vi "SetRelativePositionUm.vi"(8 "error in (no error)":errorcluster, 9 "RelativeMoveum":dbl min=0.0 max=200.0, 10 "Stage Label":string, 11 "Stage_MadCityLabMicro in":refnum<class "Stage_MadCityLabMicro.lvclass">) -> (0 "error out":errorcluster, 3 "Stage_MadCityLabMicro out":refnum<class "Stage_MadCityLabMicro.lvclass">)   [LabVIEW 2020, in "Stage_MadCityLabMicro.lvlib" / "Stage_MadCityLabMicro.lvclass"]
uses:
  Stage_MadCityLabMicro.lvclass
  Stage_MadCityLabMicro.lvclass/Stage_MadCityLabMicro.ctl
  Hardware Abstraction Layer/Component/Stage/Stage/Stage.lvclass
  Dependency/MicroDrive.dll
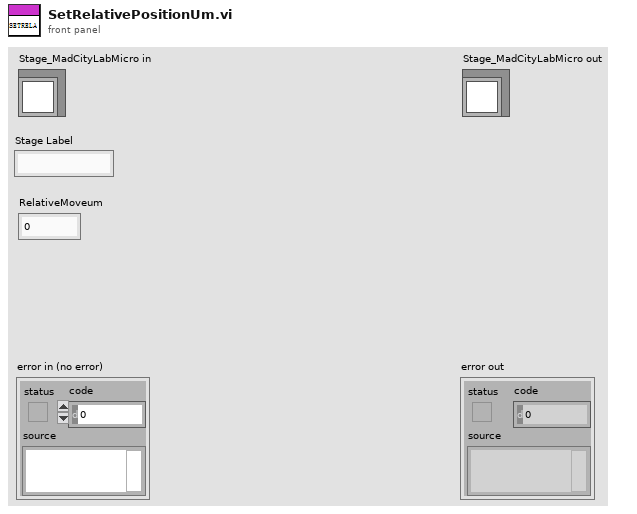
[diagram p1: front panel]
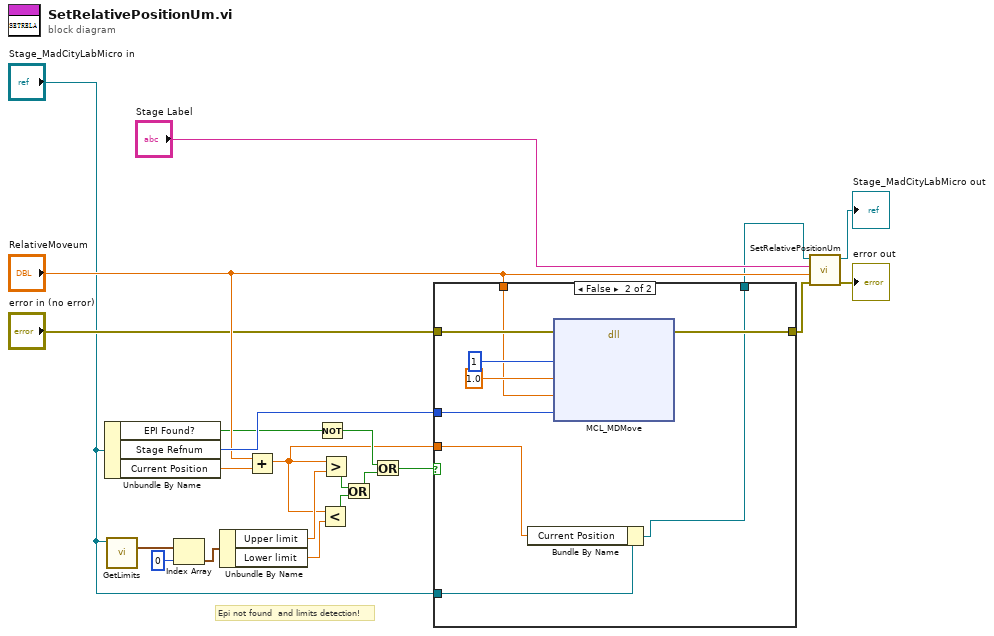
[diagram p0: block diagram]
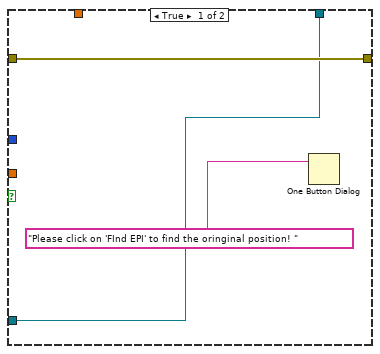
[diagram p2: hidden frame]
diagram:
  # "Epi not found  and limits detection!"
  n1 = Unbundle By Name("Stage_MadCityLabMicro in") -> ("EPI Found?"=w6:bool, "Stage Refnum"=w18:i32, "Current Position"=w12:dbl)
  n2 = call-dynamic "GetLimits.vi"("Stage in"="Stage_MadCityLabMicro in") -> ("Limits"=w14:cluster{"Upper limit":dbl, "Lower limit":dbl}[])  [unwired: 8 in, 2 out]
  n3 = Index Array(array=w14, index=0) -> (element=w15:cluster{"Upper limit":dbl, "Lower limit":dbl})
  n4 = Unbundle By Name(w15) -> ("Upper limit"=w11:dbl, "Lower limit"=w10:dbl)
  n5 = Add(x="RelativeMoveum", y=w12) -> (x+y=w3:dbl)
  n6 = Not(x=w6) -> (.not. x?=w5:bool)
  n7 = Less?(x=w3, y=w10) -> (x < y?=w8:bool)
  n8 = Greater?(x=w3, y=w11) -> (0:w9:bool)
  n9 = Or(x=w9, y=w8) -> (x .or. y?=w7:bool)
  n10 = Or(x=w5, y=w7) -> (x .or. y?=w4:bool)
  n11 = case shown="False" w4 {
    tunnel: [w25 w34] -> w19
    tunnel: w18 -> [_ w33]
    tunnel: "RelativeMoveum" -> [_ w29]
    tunnel: "error in (no error)" -> [w25 w30]
    tunnel: w3 -> [_ w27]
    tunnel: "Stage_MadCityLabMicro in" -> [w23 w28]
    tunnel: [w23 w26] -> w1
    frame True {
      n12 = One Button Dialog(message="Please click on 'FInd EPI' to find the oringinal position! ") -> ()  [unwired: 1 in, 1 out]
    }
    frame False {
      n13 = Bundle By Name(cluster=w28, "Current Position"=w27) -> (w26:refnum<class "Stage_MadCityLabMicro.lvclass">)
      n14 = dll-call lib="E:/Development/DevHardSoftware/MicroscopyFramework/Model/Hardware Layer/Real Hardware/Stage_MadCityLabMicro/Stage_MadCityLabMicro/Dependency/MicroDrive.dll" fn="MCL_MDMove"(error in=w30, "axis"=1, "velocity"=1.0, "distance"=w29, "handle"=w33) -> (error out=w34:errorcluster)  [unwired: 5 in, 3 out]
    }
  }
  n15 = call-parent "SetRelativePositionUm.vi"("error in (no error)"=w19, "RelativeMoveum"="RelativeMoveum", "Stage Label"="Stage Label", "Stage in"=w1) -> ("error out"=→"error out":errorcluster, "Stage out"=→"Stage_MadCityLabMicro out":refnum<class "Stage_MadCityLabMicro.lvclass">)  [unwired: 6 in]
